vi "speed_threshold.vi"(11 "SPEED IN":dbl) -> (3 "SPEED OUT":dbl)   [LabVIEW 2019]
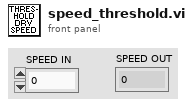
[diagram p1: front panel]
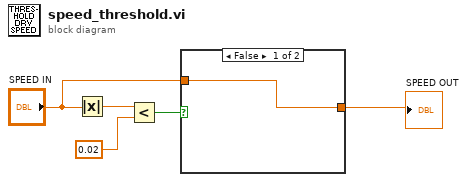
[diagram p0: block diagram]
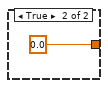
[diagram p2: hidden frame]
diagram:
  n1 = Absolute Value(x="SPEED IN") -> (abs(x)=w5:dbl)
  n2 = Less?(x=w5, y=0.02) -> (x < y?=w3:bool)
  n3 = case shown="False" w3 {
    tunnel: [w6 0.0] -> w2
    tunnel: "SPEED IN" -> [w6 _]
    frame False {
    }
    frame True {
    }
  }
  "SPEED OUT" <- w2
